vi "Read or Create I32.vi"(7 "key":string, 8 "error in (no error)":errorcluster, 9 "default value":i32, 10 "refnum":T1, 11 "Process in":refnum<class "Process.lvclass">) -> (0 "error out":errorcluster, 1 "value":i32, 2 "refnum out":T1, 3 "Process out":refnum<class "Process.lvclass">)   [LabVIEW 2020, in "Configuration File.lvlib"]
doc: "High-level function for reading configuration file data from process class."
uses:
  Configuration File.lvlib
  Process Classes/Process/Process.lvclass
  <vilib>/Utility/config.llb/NI_LVConfig.lvlib
  <vilib>/Utility/config.llb/Read Key (I32).vi
  <vilib>/Utility/config.llb/Write Key (I32).vi
  <vilib>/Utility/config.llb/Config Data RefNum.ctl
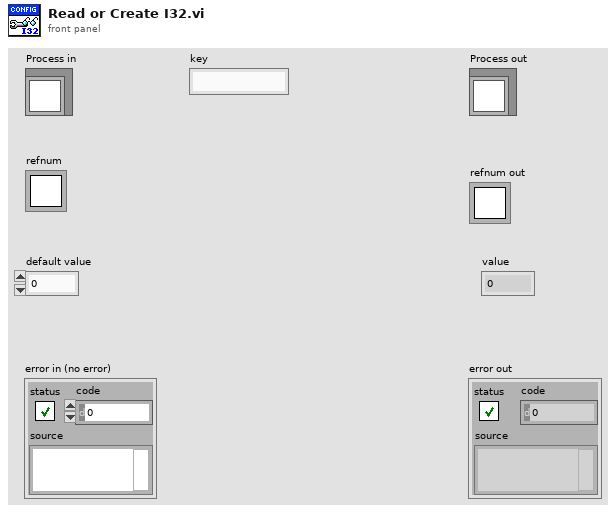
[diagram p1: front panel]
types:
  T1 = typedef "NI_LVConfig.lvlib/Config Data RefNum.ctl" = refnum<k1>
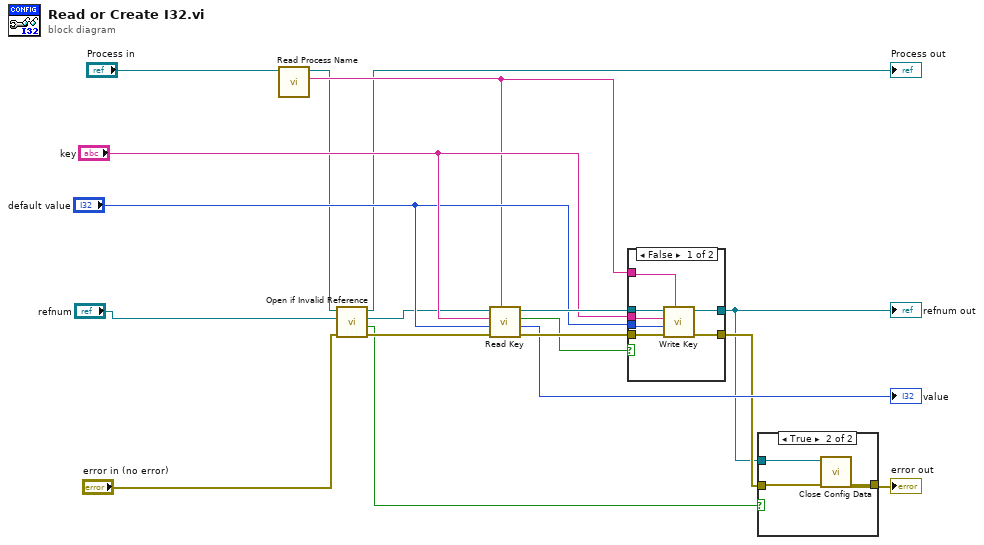
[diagram p0: block diagram]
diagram:
  n1 = call "Read Process Name.vi"("Process In"="Process in") -> ("Process Name"=w12:string, "Process Out"=w10:refnum<class "Process.lvclass">)  [unwired: 9 in]
  n2 = call "Open if Invalid Reference.vi"("error in (no error)"="error in (no error)", "refnum"="refnum", "Process in"=w10) -> ("error out"=w8:errorcluster, "File opened?"=w2:bool, "refnum out"=w6:T1, "Process out"=→"Process out":refnum<class "Process.lvclass">)  [unwired: 5 in]
  n3 = call-poly <vilib>:"Read Key.vi"("section"=w12, "error in (no error)"=w8, "default value"="default value", "key"="key", "refnum"=w6) -> ("error out"=w16:errorcluster, "value"=→"value":i32, "found?"=w15:bool, "refnum out"=w17:T1)  [unwired: 3 in]
  n4 = case shown="False" w15 {
    tunnel: w17 -> [w25 w27]
    tunnel: w16 -> [w24 w26]
    tunnel: [w23 w27] -> w3
    tunnel: [w22 w26] -> w4
    tunnel: "key" -> [w21 _]
    tunnel: "default value" -> [w20 _]
    tunnel: w12 -> [w19 _]
    frame False {
      n5 = call-poly <vilib>:"Write Key.vi"("section"=w19, "error in (no error)"=w24, "value"=w20, "key"=w21, "refnum"=w25) -> ("error out"=w22:errorcluster, "refnum out"=w23:T1)  [unwired: 4 in, 1 out]
    }
    frame True {
    }
  }
  "refnum out" <- w3
  n6 = case shown="True" w2 {
    tunnel: w3 -> [_ w31]
    tunnel: w4 -> [w28 w30]
    tunnel: [w28 w29] -> w5
    frame False {
    }
    frame True {
      n7 = call <vilib>:"Close Config Data.vi"("error in (no error)"=w30, "refnum"=w31) -> ("error out"=w29:errorcluster)  [unwired: 8 in, 1 out]
    }
  }
  "error out" <- w5
